vi "MySetMagneticField (SubVI).vi"(0 "VISA Refnum in":refnum<visa-resource-name>, 1 "Maximum trial":i32=2, 2 "Hold at end?":bool=TRUE, 3 "Max rate":dbl=0.1, 5 "Target B (T)":dbl, 7 "Present B (T)":dbl, 9 "Sweep rate":dbl=0.1, 11 "error in (no error)":errorcluster, 12 "Timeout (s) in":u16=60, 13 "Precision":dbl=0.001, 14 "Default rate":dbl=0.05) -> (4 "VISA Refnum out":refnum<visa-resource-name>, 6 "Final B (T)":dbl, 15 "error out":errorcluster)   [LabVIEW 2025, in "MyTriton.lvlib"]
uses:
  MyTriton.lvlib
  Cryo/Cryo.lvlib
panel:
  out "Last B read from VRM":dbl
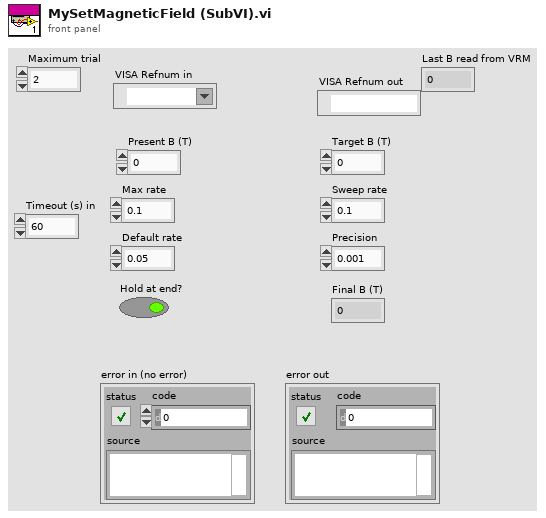
[diagram p1: front panel]
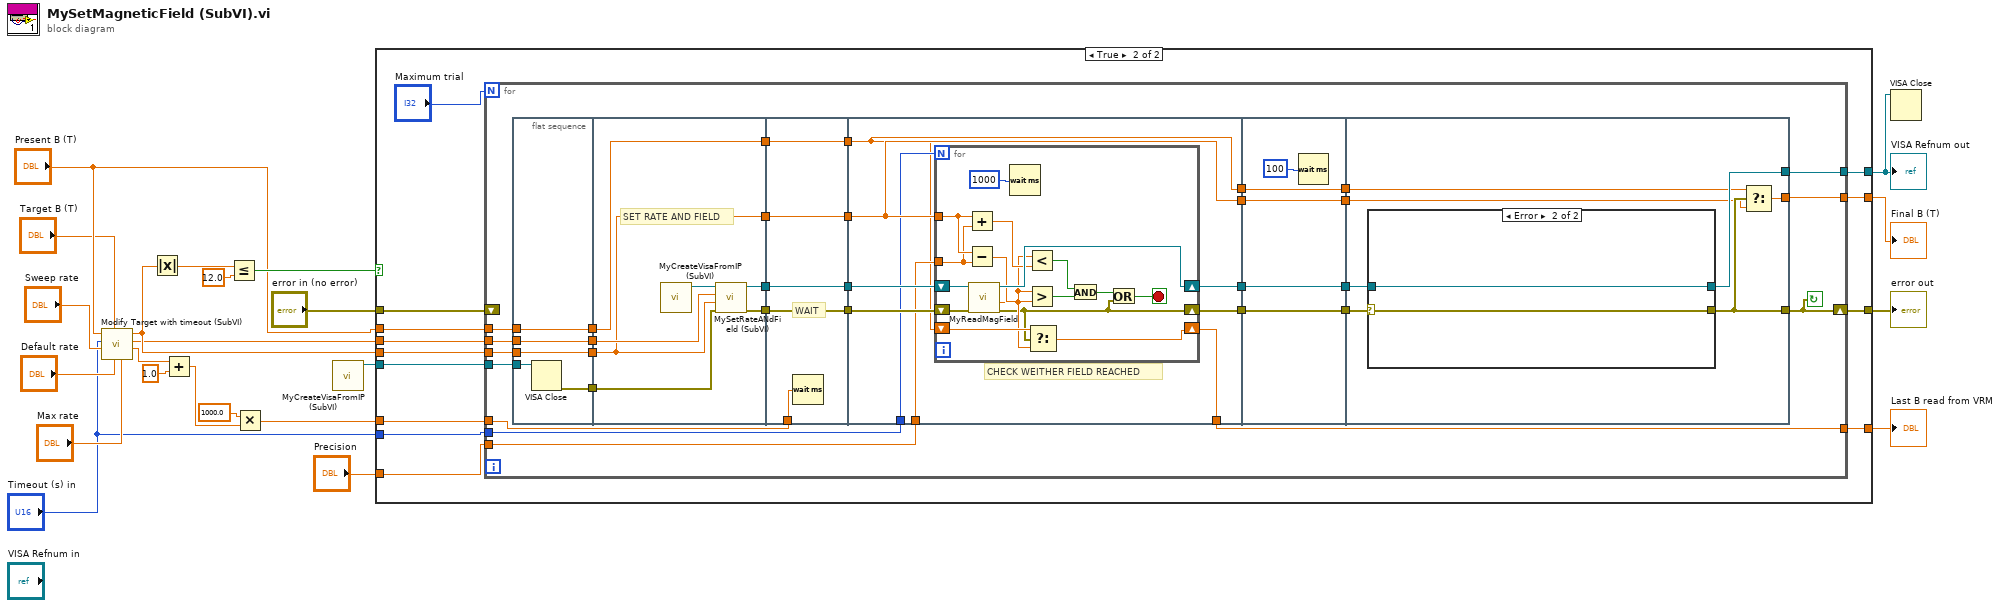
[diagram p0: block diagram]
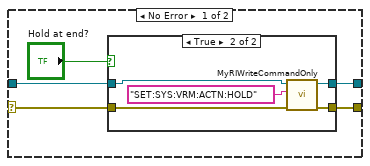
[diagram p3: hidden frame]
diagram:
  n1 = call "Modify Target with timeout (SubVI).vi"("Max Rate"="Max rate", "Default Rate"="Default rate", "Target in"="Target B (T)", "Sweep rate in"="Sweep rate", "Timeout (s) in"="Timeout (s) in", "Present value"="Present B (T)") -> ("Timeout (s) out"=w3:dbl, "Sweep rate out"=w8:dbl, "Target out"=w9:dbl)  [unwired: 3 in]
  n2 = Absolute Value(x=w9) -> (abs(x)=w22:dbl)
  n3 = Add(x=w3, y=1.0) -> (x+y=w6:dbl)
  n4 = Less Or Equal?(x=w22, y=12.0) -> (x <= y?=w20:bool)
  n5 = Multiply(x=1000.0, y=w6) -> (x*y=w4:dbl)
  n6 = call "MyCreateVisaFromIP (SubVI).vi"() -> ("VISA Refnum out"=w17:refnum<visa-resource-name>)  [unwired: 11 in]
  n7 = case shown="True" w20 {
    tunnel: "error in (no error)" -> [w25 w39]
    tunnel: w17 -> [w26 w38]
    tunnel: [w26 w34] -> w18
    tunnel: w8 -> [_ w37]
    tunnel: w9 -> [_ w36]
    tunnel: [w25 w35] -> w16
    tunnel: [w24 w30] -> w19
    tunnel: "Present B (T)" -> [w24 w33]
    tunnel: "Precision" -> [_ w32]
    tunnel: w4 -> [_ w29]
    tunnel: "Timeout (s) in" -> [_ w28]
    tunnel: [w24 w27] -> w1
    frame False {
    }
    frame True {
      n8 = for {
        N: "Maximum trial" -> [_]
        tunnel: w38 -> [w52]
        tunnel: w37 -> [w51]
        tunnel: w36 -> [w50]
        tunnel: [w49] -> w34
        tunnel: w32 -> [w47]
        shift-right: [w46] -> w35
        shift-left: w39 -> [_]
        tunnel: w29 -> [w44]
        tunnel: w28 -> [w43]
        tunnel: w33 -> [w48]
        tunnel: [w45] -> w30
        tunnel: [w40] -> w27
        stop <- w46 continue-if-true
        n9 = flat-sequence {
          tunnel: w48 -> [w73]
          tunnel: w50 -> [w74]
          tunnel: w51 -> [w75]
          tunnel: w52 -> [w72]
          tunnel: [w71] -> w70
          tunnel: [w75] -> w69
          tunnel: [w74] -> w68
          tunnel: [w73] -> w67
          tunnel: [w81] -> w65
          tunnel: [w80] -> w66
          tunnel: [w78] -> w64
          tunnel: [w77] -> w63
          tunnel: w70 -> [w82]
          tunnel: w69 -> [w79]
          tunnel: w68 -> [w78]
          tunnel: w67 -> [w77]
          tunnel: w66 -> [w87]
          tunnel: [w87] -> w62
          tunnel: w65 -> [w86]
          tunnel: [w86] -> w61
          tunnel: w64 -> [w84]
          tunnel: [w84] -> w60
          tunnel: w63 -> [w85]
          tunnel: [w85] -> w59
          tunnel: w44 -> [w83]
          tunnel: [w94] -> w58
          tunnel: [w93] -> w57
          tunnel: w62 -> [w96]
          tunnel: w61 -> [w95]
          tunnel: w60 -> [w92]
          tunnel: [w92] -> w56
          tunnel: w59 -> [w89]
          tunnel: w47 -> [w91]
          tunnel: w43 -> [w90]
          tunnel: [w89] -> w41
          tunnel: [w88] -> w40
          tunnel: w58 -> [w117]
          tunnel: [w117] -> w55
          tunnel: w57 -> [w116]
          tunnel: [w116] -> w54
          tunnel: [w114] -> w53
          tunnel: w56 -> [w114]
          tunnel: [w113] -> w42
          tunnel: w41 -> [w113]
          tunnel: w55 -> [w124]
          tunnel: w54 -> [w123]
          tunnel: [w121] -> w46
          tunnel: [w122] -> w49
          tunnel: w53 -> [w120]
          tunnel: [w119] -> w45
          tunnel: w42 -> [w118]
          frame #0 {
            n10 = VISA Close(VISA resource name=w72) -> (error out=w71:errorcluster)  [unwired: 1 in]
          }
          frame #1 {
            # "SET RATE AND FIELD"
            n11 = call "MyCreateVisaFromIP (SubVI).vi"() -> ("VISA Refnum out"=w76:refnum<visa-resource-name>)  [unwired: 11 in]
            n12 = call "MySetRateANdField (SubVI).vi"("error in (no error)"=w82, "Target B (T)"=w78, "Sweep rate"=w79, "VISA Refnum in"=w76) -> ("error out"=w81:errorcluster, "VISA Refnum out"=w80:refnum<visa-resource-name>)  [unwired: 6 in]
          }
          frame #2 {
            # "WAIT"
            n13 = Wait (ms)(milliseconds to wait=w83) -> ()  [unwired: 1 out]
          }
          frame #3 {
            # "CHECK WEITHER FIELD REACHED"
            n14 = for {
              N: w90 -> [_]
              shift-right: [w110] -> w94
              shift-left: w96 -> [w112]
              shift-right: [w99] -> w93
              shift-left: w95 -> [w111]
              tunnel: w92 -> [w108]
              shift-right: [w101] -> w88
              shift-left: w89 -> [w103]
              tunnel: w91 -> [w97]
              stop <- w98 stop-if-true
              n15 = Add(x=w108, y=w97) -> (x+y=w109:dbl)
              n16 = Subtract(x=w108, y=w97) -> (x-y=w107:dbl)
              n17 = call "MyReadMagField.vi"("error in (no error)"=w111, "VISA resource name in"=w112) -> ("error out"=w99:errorcluster, "B"=w102:dbl, "VISA resource name out"=w110:refnum<visa-resource-name>)  [unwired: 7 in]
              n18 = Wait (ms)(milliseconds to wait=u32 1000) -> ()  [unwired: 1 out]
              n19 = Less?(x=w102, y=w109) -> (x < y?=w106:bool)
              n20 = Greater?(x=w102, y=w107) -> (0:w105:bool)
              n21 = Select(t=w103, s=w99, f=w102) -> (s? t:f=w101:dbl)
              n22 = And(x=w106, y=w105) -> (x .and. y?=w100:bool)
              n23 = Or(x=w100, y=w99) -> (x .or. y?=w98:bool)
            }
          }
          frame #4 {
            n24 = Wait (ms)(milliseconds to wait=u32 100) -> ()  [unwired: 1 out]
          }
          frame #5 {
            n25 = case shown="Error" w123 {
              selector: w123 -> [w128 w138]
              tunnel: w124 -> [w129 w137]
              tunnel: [w126 w137] -> w122
              tunnel: [w127 w138] -> w121
              frame No Error {
                n26 = case shown="True" "Hold at end?" {
                  tunnel: w129 -> [w131 w135]
                  tunnel: w128 -> [w130 w134]
                  tunnel: [w130 w133] -> w127
                  tunnel: [w131 w132] -> w126
                  frame False {
                  }
                  frame True {
                    n27 = call "MyRIWriteCommandOnly.vi"("error in (no error)"=w134, "Command"="SET:SYS:VRM:ACTN:HOLD", "VISA resource name in"=w135) -> ("error out"=w133:errorcluster, "VISA resource name out"=w132:refnum<visa-resource-name>)  [unwired: 7 in]
                  }
                }
              }
              frame Error {
              }
            }
            n28 = Select(t=w118, s=w121, f=w120) -> (s? t:f=w119:dbl)
          }
        }
      }
    }
  }
  "error out" <- w16
  "VISA Refnum out" <- w18
  "Final B (T)" <- w19
  "Last B read from VRM" <- w1
  n29 = VISA Close(VISA resource name=w18) -> ()  [unwired: 1 in, 1 out]
